vi "HAL camera get temp - SubVI.vi"(0 "Cooling status In":T1) -> (1 "Error?":bool, 2 "Cooling status Out":T1, 3 "Current temperature":i32)   [LabVIEW 2014]
uses:
  ATMCD32D.DLL
  Glimpse-master/Microscope plugins/ixon camera/HAL cooling status.ctt
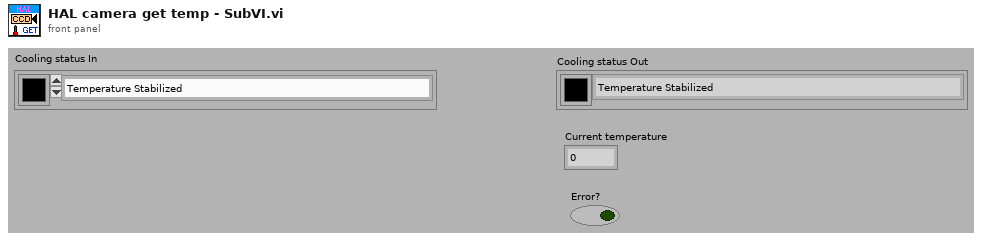
[diagram p1: front panel]
types:
  T1 = typedef "HAL cooling status.ctt" = cluster{"Color Box":u32, "Cooling Status":enum16{"Temperature Stabilized", "Waiting to Stabilize Temperature", "Cooling is Turned Off", "Have not yet Reached Set Temperature"}}
  T2 = enum16{"Temperature Stabilized", "Waiting to Stabilize Temperature", "Cooling is Turned Off", "Have not yet Reached Set Temperature"}
  T3 = enum16{"Temperature Stabilized", "Waiting to Stabilize Temperature", "Cooling is Turned Off"}
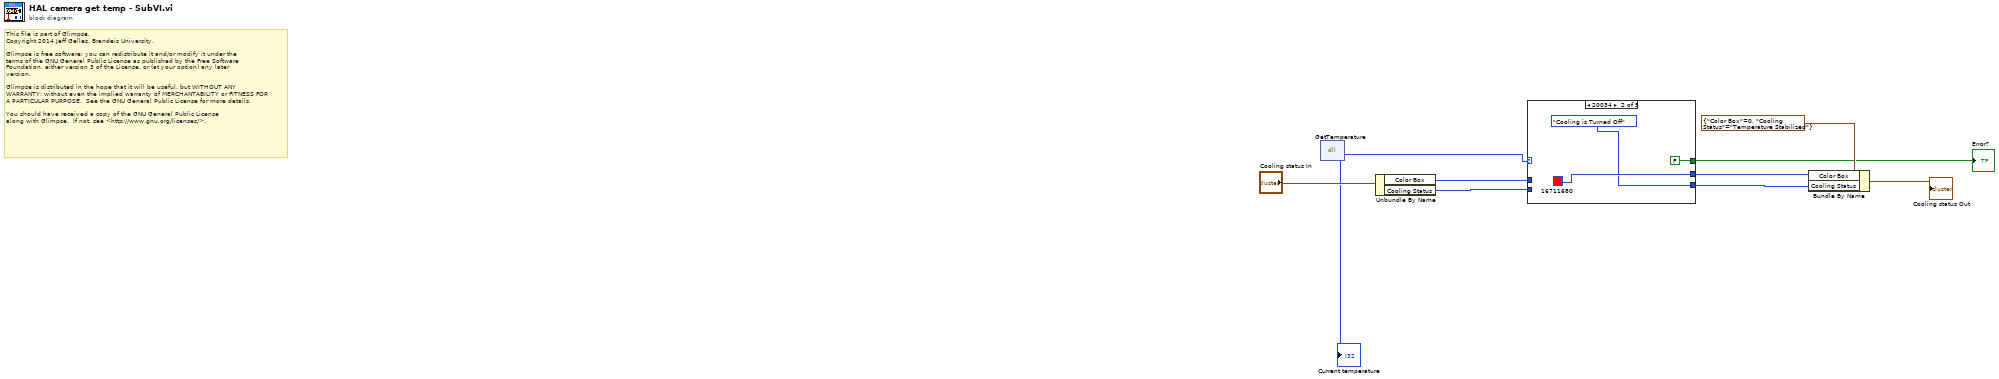
[diagram p0: block diagram]
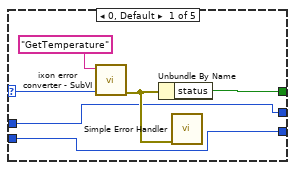
[diagram p2: hidden frame]
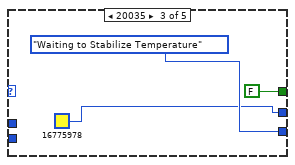
[diagram p3: hidden frame]
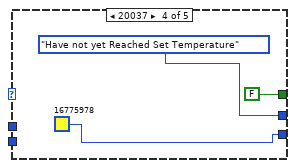
[diagram p4: hidden frame]
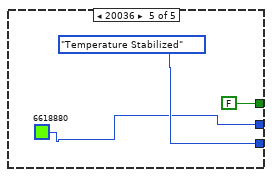
[diagram p5: hidden frame]
diagram:
  # "This file is part of Glimpse. \nCopyright 2014 Jeff Gelles, Brandeis University.    \n\nGlimpse is free software: you can redistribute it and/or modify it under the \nterms of the GNU General Public License as published by the Free Software \nFoundation, either version 3 of the License, or (at your option) any later \nversion.\n\nGlimpse is distributed in the hope that it will be useful, but WITHOUT ANY \nWARRANTY; without even the implied warranty of MERCHANTABILITY or FITNESS FOR \nA PARTICULAR PURPOSE.  See the GNU General Public License for more details.\n\nYou should have received a copy of the GNU General Public License\nalong with Glimpse.  If not, see <http://www.gnu.org/licenses/>."
  n1 = dll-call lib="ATMCD32D.DLL" fn="GetTemperature"() -> (w1:u32, →"Current temperature":i32)  [unwired: 3 in, 3 out]
  n2 = Unbundle By Name("Cooling status In") -> ("Color Box"=w9:u32, "Cooling Status"=w10:T2)
  n3 = case shown="20034" w1 {
    selector: w1 -> [w16 _ _ _ _]
    tunnel: [w14 FALSE ("status") FALSE ("status") FALSE ("status") FALSE ("status")] -> w3
    tunnel: [w12 u32 16711680 u32 16775978 T2."Have not yet Reached Set Temperature" ("Cooling Status") u32 6618880] -> w6
    tunnel: [w11 T3."Cooling is Turned Off" ("Cooling Status") T3."Waiting to Stabilize Temperature" ("Cooling Status") u32 16775978 T3."Temperature Stabilized" ("Cooling Status")] -> w7
    tunnel: w9 -> [w12 _ _ _ _]
    tunnel: w10 -> [w11 _ _ _ _]
    frame 0, Default {
      n4 = call "ixon error converter - SubVI.vi"("Andor error code"=w16, "source"="GetTemperature") -> ("error out"=w13:errorcluster)  [unwired: 5 in]
      n5 = Unbundle By Name(w13) -> ("status"=w14:bool)
      n6 = call <vilib>:"Simple Error Handler.vi"("error in (no error)"=w13) -> ()  [unwired: 1 in, 8 out]
    }
    frame 20034 {
    }
    frame 20035 {
    }
    frame 20037 {
    }
    frame 20036 {
    }
  }
  "Error?" <- w3
  n7 = Bundle By Name(cluster=T1 {"Color Box"=0, "Cooling Status"=enum."Temperature Stabilized"} ("Cooling status"), "Color Box"=w6, "Cooling Status"=w7) -> (→"Cooling status Out":T1)
